vi "pop next connection.vi"(8 "error in":errorcluster, 11 "conn creator":u64) -> (0 "error out":errorcluster, 3 "connection handle":u64)   [LabVIEW 2016, in "async tls dl.lvlib"]
uses:
  async tls dl.lvlib
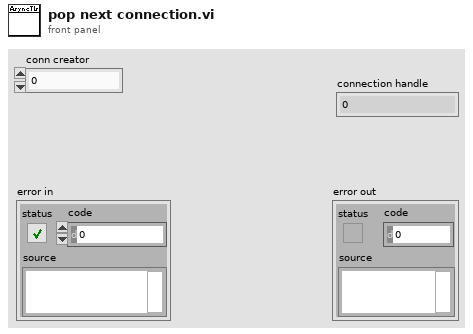
[diagram p1: front panel]
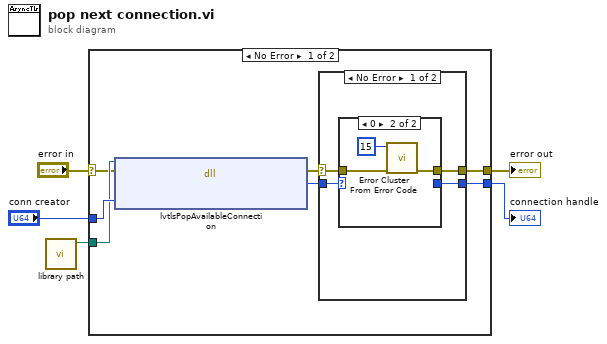
[diagram p0: block diagram]
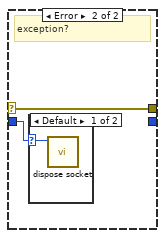
[diagram p3: hidden frame]
diagram:
  n1 = call "library path.vi"() -> ("path"=w4:path)  [unwired: 11 in]
  n2 = case shown="No Error" "error in" {
    selector: "error in" -> [w9 w25]
    tunnel: "conn creator" -> [w11 _]
    tunnel: w4 -> [w10 _]
    tunnel: [w8 w25] -> w2
    tunnel: [w6 _] -> w1
    frame No Error {
      n3 = dll-call lib="C:/Users/IEUser/Desktop/libasynclvtls/lvasynctls.dll" fn="lvtlsPopAvailableConnection" ("lvasynctls.dll:lvtlsDisposeClientConnector")(path in=w10, error in=w9, "connCreator"=w11) -> (error out=w12:errorcluster, "connection"=w7:u64)  [unwired: 2 in, 1 out]
      n4 = case shown="No Error" w12 {
        selector: w12 -> [w16 w23]
        tunnel: [w15 w23] -> w8
        tunnel: w7 -> [w14 w22]
        tunnel: [w13 _] -> w6
        frame No Error {
          n5 = case shown="0" w14 {
            selector: w14 -> [w17 _]
            tunnel: w16 -> [w18 w21]
            tunnel: [w18 w20] -> w15
            tunnel: [w17 _] -> w13
            frame Default {
            }
            frame 0 {
              n6 = call <vilib>:"Error Cluster From Error Code.vi"("error in (no error)"=w21, "error code (0)"=15) -> ("error out"=w20:errorcluster)  [unwired: 7 in]
            }
          }
        }
        frame Error {
          # "exception?"
          n7 = case shown="Default" w22 {
            selector: w22 -> [w24 _]
            frame Default {
              n8 = call "dispose socket.vi"("socket"=w24) -> ()  [unwired: 10 in, 1 out]
            }
            frame 0 {
            }
          }
        }
      }
    }
    frame Error {
    }
  }
  "error out" <- w2
  "connection handle" <- w1
